vi "Set Line Width.vi"(8 "error in (no error)":errorcluster, 10 "Value":string, 11 "GraphChart in":refnum<vi>) -> (0 "error out":errorcluster)   [LabVIEW 2019, in "LSS.lvlib"]
doc: "Apply the desired color properties to either a Waveform Graph or Chart. Though LabVIEW uses two different property nodes to do this set, with LSS the same properties can be applied to both and this VI will determine which property node to use.\n\n<b>Inputs:</b>\n<b>GraphChart in</b> - Reference to the graph that will be set.\n<b>Value</b> - Value of the plot reference number and color.\n<b>Error In</b> - Standard Error in terminal.\n\n<b>Outputs:</b>\n<b>Error out</b> - Standard Error out terminal."
uses:
  LSS.lvlib
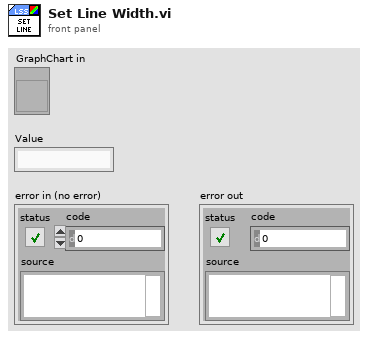
[diagram p1: front panel]
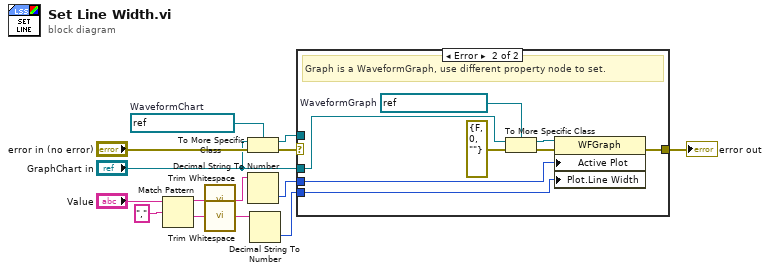
[diagram p0: block diagram]
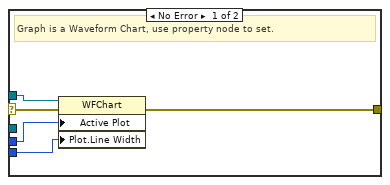
[diagram p2: hidden frame]
diagram:
  w8 = refnum<vi> refnum  # WaveformChart
  n1 = Match Pattern(string="Value", regular expression=",") -> (before substring=w11:string, after substring=w9:string)  [unwired: 1 in, 2 out]
  n2 = call <vilib>:"Trim Whitespace.vi"("string"=w11) -> ("trimmed string"=w13:string)  [unwired: 1 in]
  n3 = call <vilib>:"Trim Whitespace.vi"("string"=w9) -> ("trimmed string"=w2:string)  [unwired: 1 in]
  n4 = To More Specific Class(target class=w8, reference="GraphChart in", error in="error in (no error)") -> (specific class reference=w7:refnum<vi>, error out=w6:errorcluster)
  n5 = Decimal String To Number(string=w13) -> (number=w4:i32)  [unwired: 2 in, 1 out]
  n6 = Decimal String To Number(string=w2) -> (number=w1:i32)  [unwired: 2 in, 1 out]
  n7 = case shown="Error" w6 {
    selector: w6 -> [w18 _]
    tunnel: w7 -> [w19 _]
    tunnel: w4 -> [w17 w24]
    tunnel: [w16 w22] -> w5
    tunnel: "GraphChart in" -> [_ w21]
    tunnel: w1 -> [w15 w20]
    frame No Error {
      # "Graph is a Waveform Chart, use property node to set."
      n8 = property class="WFChart"(reference=w19, error in=w18, "Active Plot"=w17, "Plot.Line Width"=w15) -> (error out=w16:errorcluster)  [unwired: 1 out]
    }
    frame Error {
      w27 = refnum<vi> refnum  # WaveformGraph
      # "Graph is a WaveformGraph, use different property node to set."
      n9 = To More Specific Class(target class=w27, reference=w21, error in=errorcluster {"status"=FALSE, "code"=0, "source"=""}) -> (specific class reference=w26:refnum<vi>, error out=w25:errorcluster)
      n10 = property class="WFGraph"(reference=w26, error in=w25, "Active Plot"=w24, "Plot.Line Width"=w20) -> (error out=w22:errorcluster)  [unwired: 1 out]
    }
  }
  "error out" <- w5
